vi "ViperHawk Sort Search Parameters.vi"(8 "Error In":errorcluster, 10 "Debug Search Parameters":T1, 11 "Full Message":string) -> (0 "Error Out":errorcluster, 2 "Enum":T2(ring))   [LabVIEW 2016]
uses:
  Type Definitions/ViperHawk/ViperHawk Search Control.ctl
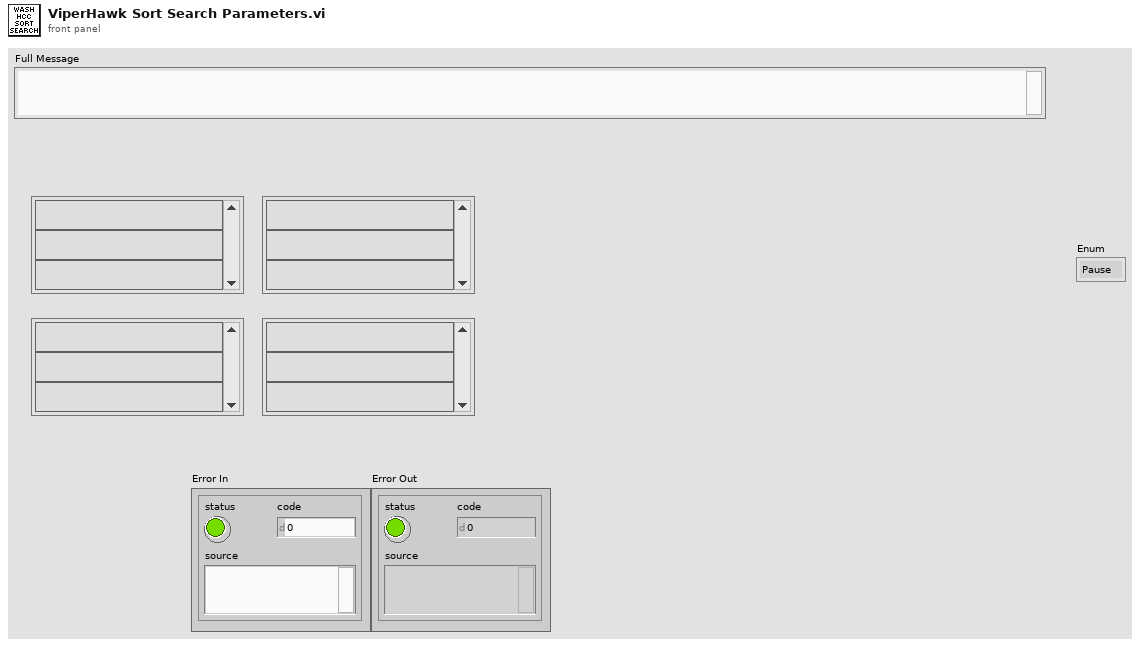
[diagram p1: front panel]
types:
  T1 = typedef "ViperHawk Search Control.ctl" = cluster{"Pause":string[], "Run":string[], "EOC":string[], "Error Codes":string[]}
  T2 = enum16{"Pause", "Run", "EOC", "Do Nothing", "Error Codes"}
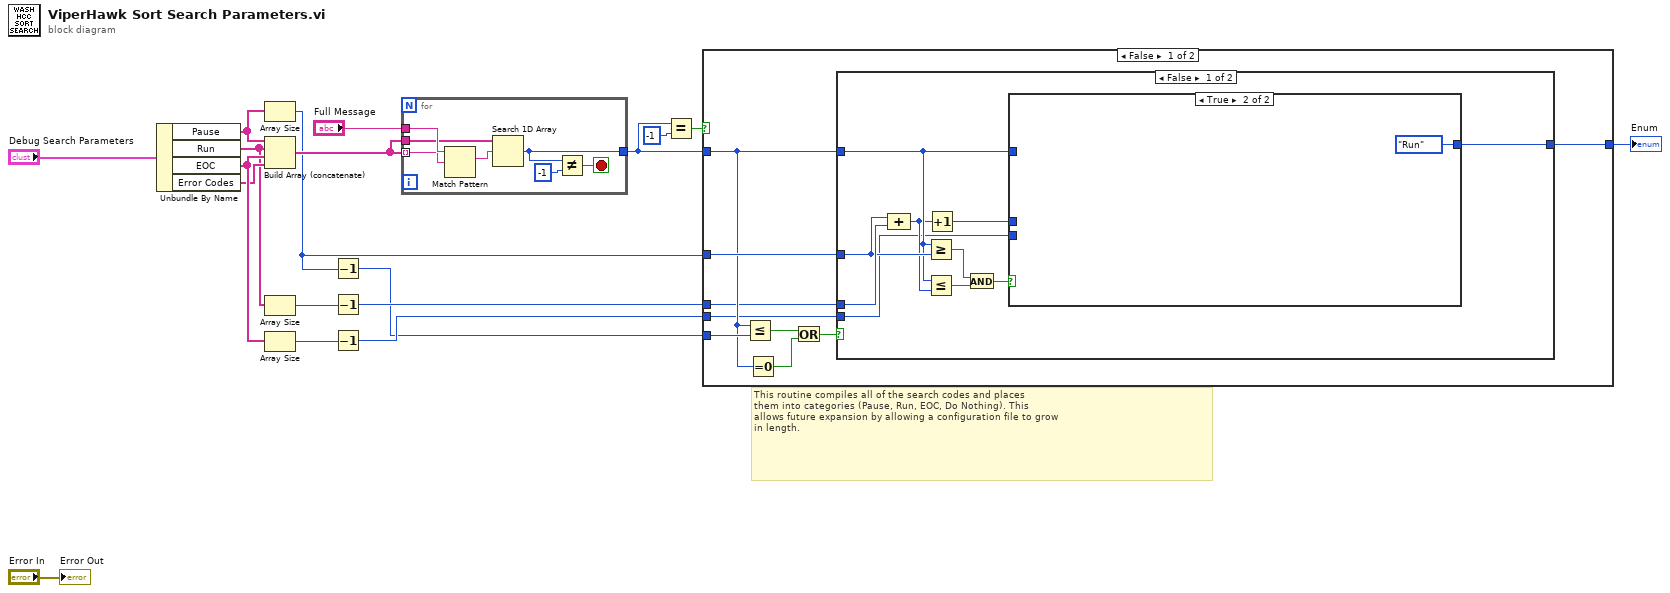
[diagram p0: block diagram]
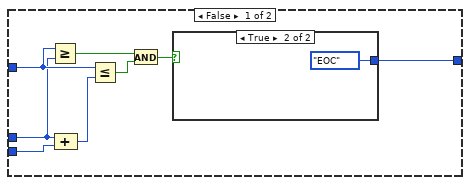
[diagram p2: hidden frame]
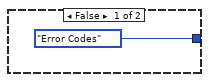
[diagram p3: hidden frame]
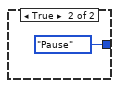
[diagram p4: hidden frame]
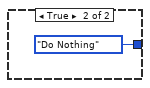
[diagram p5: hidden frame]
diagram:
  # "This routine compiles all of the search codes and places\nthem into categories (Pause, Run, EOC, Do Nothing). This \nallows future expansion by allowing a configuration file to grow\nin length."
  n1 = Unbundle By Name("Debug Search Parameters") -> ("Pause"=w4:string[], "Run"=w5:string[], "EOC"=w15:string[], "Error Codes"=w14:string[])
  n2 = Array Size(array=w4) -> (size(s)=w7:i32)
  n3 = Build Array (concatenate)(w4, w5, w15, w14) -> (w13:string[])
  n4 = Array Size(array=w5) -> (size(s)=w8:i32)
  n5 = Array Size(array=w15) -> (size(s)=w16:i32)
  n6 = Decrement(x=w7) -> (x-1=w6:i32)
  n7 = Decrement(x=w8) -> (x-1=w9:i32)
  n8 = Decrement(x=w16) -> (x-1=w17:i32)
  n9 = for {
    tunnel: w13 -> [w24] mode=indexing
    tunnel: "Full Message" -> [w25]
    tunnel: w13 -> [w23]
    tunnel: [w19] -> w10
    stop <- w20 stop-if-true
    n10 = Match Pattern(string=w25, regular expression=w24) -> (match substring=w22:string)  [unwired: 1 in, 3 out]
    n11 = Search 1D Array(1D array=w23, element=w22) -> (index of element=w19:i32)  [unwired: 1 in]
    n12 = Not Equal?(x=w19, y=-1) -> (x != y?=w20:bool)
  }
  n13 = Equal?(x=w10, y=-1) -> (x = y?=w12:bool)
  n14 = case shown="False" w12 {
    tunnel: w6 -> [w33 _]
    tunnel: w7 -> [w32 _]
    tunnel: w10 -> [w31 _]
    tunnel: w9 -> [w30 _]
    tunnel: [w29 T2."Do Nothing"] -> w18
    tunnel: w17 -> [w26 _]
    frame False {
      n15 = Less Or Equal?(x=w31, y=w33) -> (x <= y?=w28:bool)
      n16 = Equal To 0?(x=w31) -> (x = 0?=w27:bool)
      n17 = Or(x=w28, y=w27) -> (x .or. y?=w34:bool)
      n18 = case shown="False" w34 {
        tunnel: [w40 T2."Pause"] -> w29
        tunnel: w32 -> [w39 _]
        tunnel: w31 -> [w38 _]
        tunnel: w30 -> [w43 _]
        tunnel: w26 -> [w35 _]
        frame False {
          n19 = Compound Arithmetic op=ADD(w39, w43) -> (w37:i32)
          n20 = Greater Or Equal?(x=w38, y=w39) -> (x >= y?=w44:bool)
          n21 = Less Or Equal?(x=w38, y=w37) -> (x <= y?=w42:bool)
          n22 = Increment(x=w37) -> (x+1=w36:i32)
          n23 = And(x=w44, y=w42) -> (x .and. y?=w41:bool)
          n24 = case shown="True" w41 {
            tunnel: [w45 T2."Run"] -> w40
            tunnel: w38 -> [w52 _]
            tunnel: w36 -> [w51 _]
            tunnel: w35 -> [w50 _]
            frame False {
              n25 = Greater Or Equal?(x=w52, y=w51) -> (x >= y?=w48:bool)
              n26 = Compound Arithmetic op=ADD(w51, w50) -> (w49:i32)
              n27 = Less Or Equal?(x=w52, y=w49) -> (x <= y?=w47:bool)
              n28 = And(x=w48, y=w47) -> (x .and. y?=w46:bool)
              n29 = case shown="True" w46 {
                tunnel: [T2."Error Codes" T2."EOC"] -> w45
                frame False {
                }
                frame True {
                }
              }
            }
            frame True {
            }
          }
        }
        frame True {
        }
      }
    }
    frame True {
    }
  }
  "Enum" <- w18
  "Error Out" <- "Error In"
